vi "getServerParams.vi"() -> (0 "NodeId":string, 1 "ServerURL":string)   [LabVIEW 2025]
uses:
  <vilib>/Utility/config.llb/NI_LVConfig.lvlib
  <vilib>/Utility/config.llb/Read Key (String).vi
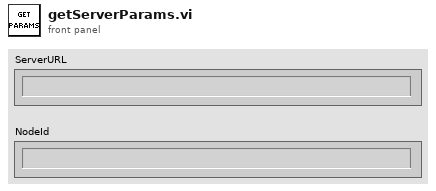
[diagram p1: front panel]
types:
  T1 = typedef "NI_LVConfig.lvlib/Config Data RefNum.ctl" = refnum<k1>
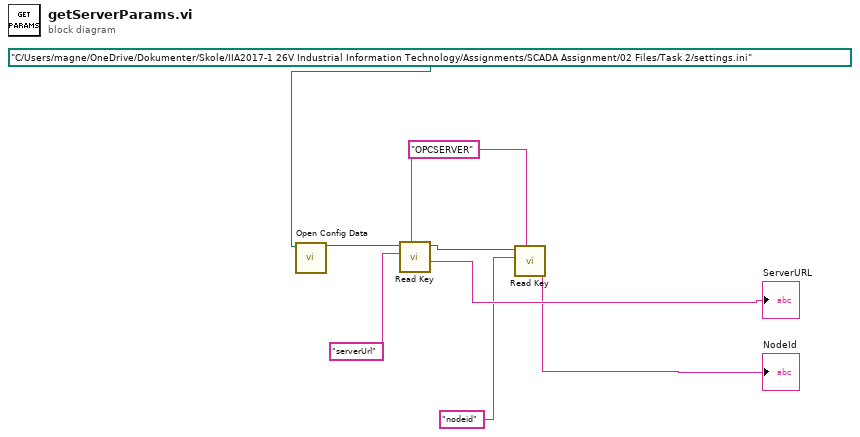
[diagram p0: block diagram]
diagram:
  w1 = "OPCSERVER" ("section")
  n1 = call <vilib>:"Open Config Data.vi"("configuration file path"=path "C:/Users/magne/OneDrive/Dokumenter/Skole/IIA2017-1 26V Industrial Information Technology/Assignments/SCADA Assignment/02 Files/Task 2/settings.ini") -> ("refnum"=w5:T1)  [unwired: 8 in, 2 out]
  n2 = call-poly <vilib>:"Read Key.vi"("section"=w1, "key"="serverUrl", "refnum"=w5) -> ("value"=→"ServerURL":string, "refnum out"=w4:T1)  [unwired: 5 in, 2 out]
  n3 = call-poly <vilib>:"Read Key.vi"("section"=w1, "key"="nodeid", "refnum"=w4) -> ("value"=→"NodeId":string)  [unwired: 5 in, 3 out]
